vi "PathPlanner_PathFinder_DoMinorALT.vi"() -> (0 "Error":bool)   [LabVIEW 2019, in "PathPlanner24.lvlib"]
doc: "Internal function. Not to be used by end users."
uses:
  PathPlanner24.lvlib
  PathPlanner_GridPosition_Equals.vi
  PathPlanner_PathFinder_GridPosToTranslation2d.vi
  PathPlanner_PathFinder_ApplyControlSmooth.vi
  PathPlanner_PathFinder_ExtractPathSub1ALT.vi
  PathPlanner_PathFinder_IsWalkable.vi
  PathPlanner_PathFinder_ApplyAnchorSmooth.vi
  <vilib>/Rock Robotics/WPI/ThirdParty/JAS_Junk/TrajLib/Translation2d_GetDistance.vi
  PathPlanner_PathFinder_Constants.vi
  <vilib>/Rock Robotics/WPI/ThirdParty/JAS_Junk/TrajLib/Translation2d_Create_DistAng.vi
  <vilib>/Rock Robotics/WPI/ThirdParty/JAS_Junk/TrajLib/Translation2d_Minus.vi
  <vilib>/Rock Robotics/WPI/ThirdParty/JAS_Junk/TrajLib/Translation2d_GetAngle.vi
  <vilib>/Rock Robotics/WPI/ThirdParty/JAS_Junk/TrajLib/Translation2d_Plus.vi
  <vilib>/Rock Robotics/WPI/ThirdParty/JAS_Junk/TrajLib/Translation2d_Create.vi
  <vilib>/Rock Robotics/WPI/ThirdParty/JAS_Junk/TrajLib/Translation2d_Times.vi
  PathPlanner_GridPosition_New.vi
  <vilib>/Rock Robotics/WPI/ThirdParty/JAS_Junk/TrajLib/Util_CalcDist.vi
  <vilib>/Rock Robotics/WPI/ThirdParty/JAS_Junk/TrajLib/Rotation2d_GetAngleCosSin.vi
  <vilib>/Rock Robotics/WPI/ThirdParty/JAS_Junk/TrajLib/Translation2d_GetXY.vi
  <vilib>/Rock Robotics/WPI/ThirdParty/JAS_Junk/TrajLib/Rotation2d_CreateXY.vi
  <vilib>/robotics/Navigation/shared/MapNode/OccupancyGridNode/NI_Robotics_OccupancyGridMapNode.lvclass
  C:/Program Files/National Instruments/LabVIEW 2019/vi.lib/robotics/Navigation/shared/MapNode/AbstractDstarNode/NI_Robotics_AbstractDstarNode.lvclass
  <vilib>/robotics/Navigation/shared/MapNode/AbstractDstarNode/NI_Robotics_AbstractDstarNode.lvclass
  C:/Program Files/National Instruments/LabVIEW 2019/vi.lib/robotics/Navigation/shared/MapNode/AbstractAstarNode/NI_Robotics_AbstractAstarNode.lvclass
  PathPlanner_PathFinder_Globals.vi
  <vilib>/robotics/Navigation/shared/WorldMap/OccupancyGridWorldMap/Get Cells in Path.vi
  <vilib>/robotics/Navigation/Anytime D Star/NI_Robotics_AnytimeDStar.lvclass
  <vilib>/robotics/Navigation/shared/WorldMap/OccupancyGridWorldMap/NI_Robotics_OccupancyGridWorldMap.lvclass
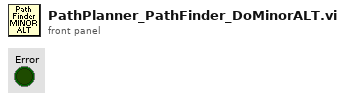
[diagram p1: front panel]
types:
  T1 = typedef "PathPlanner24.lvlib/PathPlannerFinderGridPosition.ctl" = cluster{"X":i32, "Y":i32}
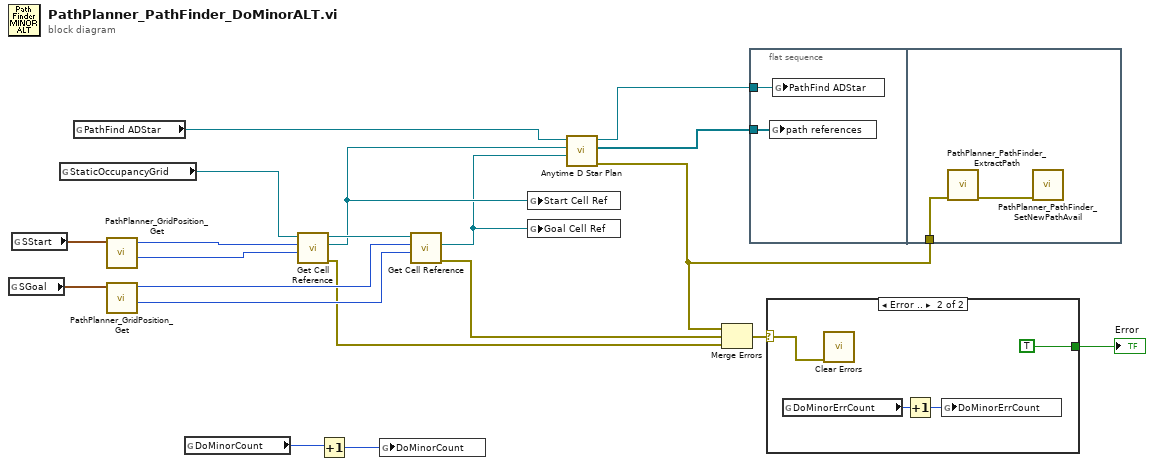
[diagram p0: block diagram]
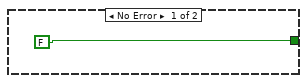
[diagram p2: hidden frame]
diagram:
  n1 = global read "PathPlanner_PathFinder_Globals.vi" "SGoal"() -> (w17:T1)
  n2 = global read "PathPlanner_PathFinder_Globals.vi" "SStart"() -> (w18:T1)
  n3 = global read "PathPlanner_PathFinder_Globals.vi" "StaticOccupancyGrid"() -> (w16:refnum<data-value>)
  n4 = global read "PathPlanner_PathFinder_Globals.vi" "PathFind ADStar"() -> (w10:refnum<class "NI_Robotics_AnytimeDStar.lvclass">)
  n5 = call "PathPlanner_GridPosition_Get.vi"("GridPosition"=w18) -> ("Int Y"=w13:i32, "Int X"=w14:i32)  [unwired: 9 in]
  n6 = call "PathPlanner_GridPosition_Get.vi"("GridPosition"=w17) -> ("Int Y"=w11:i32, "Int X"=w12:i32)  [unwired: 9 in]
  n7 = global read "PathPlanner_PathFinder_Globals.vi" "DoMinorCount"() -> (w20:i64)
  n8 = call <vilib>:"Get Cell Reference.vi"("y"=w13, "x"=w14, "map reference in"=w16) -> ("error out"=w3:errorcluster, "cell reference"=w8:refnum<data-value>, "map reference out"=w15:refnum<data-value>)  [unwired: 5 in, 1 out]
  n9 = Increment(x=w20) -> (x+1=w19:i64)
  n10 = global write "PathPlanner_PathFinder_Globals.vi" "DoMinorCount"(w19) -> ()
  n11 = call <vilib>:"Get Cell Reference.vi"("y"=w11, "x"=w12, "map reference in"=w15) -> ("error out"=w4:errorcluster, "cell reference"=w7:refnum<data-value>)  [unwired: 5 in, 2 out]
  n12 = global write "PathPlanner_PathFinder_Globals.vi" "Start Cell Ref"(w8) -> ()
  n13 = global write "PathPlanner_PathFinder_Globals.vi" "Goal Cell Ref"(w7) -> ()
  n14 = call <vilib>:"Anytime D Star Plan.vi"("new goal reference"=w7, "current reference"=w8, "Anytime D* in"=w10) -> ("error out"=w1:errorcluster, "path references"=w2:refnum<data-value>[], "Anytime D* out"=w9:refnum<class "NI_Robotics_AnytimeDStar.lvclass">)  [unwired: 4 in, 2 out]
  n15 = Merge Errors(w1, w4, w3) -> (w6:errorcluster)
  n16 = flat-sequence {
    tunnel: w9 -> [w22]
    tunnel: w2 -> [w21]
    tunnel: w1 -> [w23]
    frame #0 {
      n17 = global write "PathPlanner_PathFinder_Globals.vi" "path references"(w21) -> ()
      n18 = global write "PathPlanner_PathFinder_Globals.vi" "PathFind ADStar"(w22) -> ()
    }
    frame #1 {
      n19 = call "PathPlanner_PathFinder_ExtractPath.vi"("error in (no error)"=w23) -> ("error out"=w24:errorcluster)  [unwired: 10 in]
      n20 = call "PathPlanner_PathFinder_SetNewPathAvail.vi"("error in (no error)"=w24) -> ()  [unwired: 10 in, 1 out]
    }
  }
  n21 = case shown="Error .." w6 {
    selector: w6 -> [_ w26]
    tunnel: [FALSE TRUE] -> w5
    frame No Error {
    }
    frame Error {
      n22 = global read "PathPlanner_PathFinder_Globals.vi" "DoMinorErrCount"() -> (w28:i64)
      n23 = call <vilib>:"Clear Errors.vi"("error in (no error)"=w26) -> ()  [unwired: 5 in, 2 out]
      n24 = Increment(x=w28) -> (x+1=w27:i64)
      n25 = global write "PathPlanner_PathFinder_Globals.vi" "DoMinorErrCount"(w27) -> ()
    }
  }
  "Error" <- w5
